vi "SV TDMS Write Y Properties.vi"(0 "tdms file":refnum<k34>, 1 "y-axis label":string, 2 "y-unit string":string, 5 "group name":string, 7 "channel name":string, 11 "error in (no error)":errorcluster, 12 "xchannel name":string) -> (4 "tdms file out":refnum<k34>, 6 "group name":string, 8 "channel name":string, 15 "error out":errorcluster)   [LabVIEW 2017]
uses:
  <vilib>/addons/_NISVFA/_Shared subVIs/Controls/NI Channel Properties.ctl
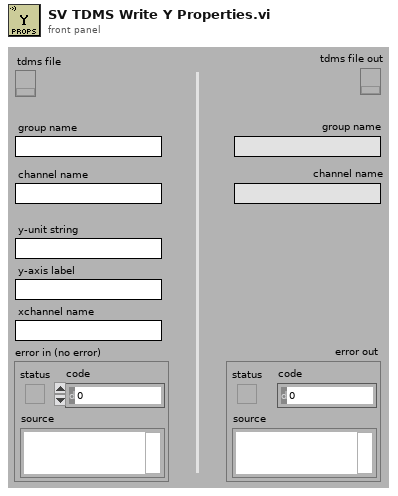
[diagram p1: front panel]
types:
  T1 = typedef "NI Channel Properties.ctl" = u16
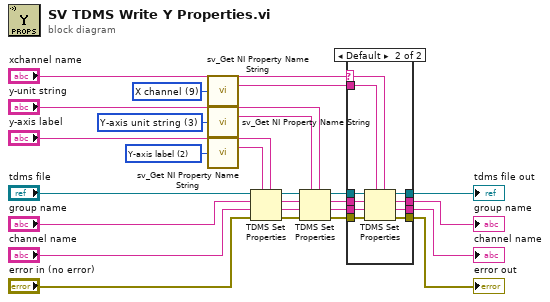
[diagram p0: block diagram]
diagram:
  w11 = T1 9 items=["Channel name", "Channel description", "Y-axis label", "Y-axis unit string", "X-axis label", "X-axis unit string", "x0", "dx", "Number of samples", "X channel", "Filter settled", "dB reference", "Window", "Window parameter", "Window size", "FFT size", "Peak units", "Spectrum type", "Magnitude scale", "Spectral density", "Sensor sensitivity (mV/EU)", "X-axis dimension", "LabVIEW datatype", "Function type", "Function subtype", "X-values"] ("property")
  w14 = T1 3 items=["Channel name", "Channel description", "Y-axis label", "Y-axis unit string", "X-axis label", "X-axis unit string", "x0", "dx", "Number of samples", "X channel", "Filter settled", "dB reference", "Window", "Window parameter", "Window size", "FFT size", "Peak units", "Spectrum type", "Magnitude scale", "Spectral density", "Sensor sensitivity (mV/EU)", "X-axis domain", "LabVIEW datatype"] ("property")
  w15 = T1 2 items=["Channel name", "Channel description", "Y-axis label", "Y-axis unit string", "X-axis label", "X-axis unit string", "x0", "dx", "Number of samples", "X channel", "Filter settled", "dB reference", "Window", "Window parameter", "Window size", "FFT size", "Peak units", "Spectrum type", "Magnitude scale", "Spectral density", "Sensor sensitivity (mV/EU)", "X-axis domain", "LabVIEW datatype"] ("property")
  n1 = call <vilib>:"sv_Get NI Property Name String.vi"("property"=w11) -> ("TDMS property name"=w10:string)  [unwired: 13 in, 1 out]
  n2 = call <vilib>:"sv_Get NI Property Name String.vi"("property"=w14) -> ("TDMS property name"=w13:string)  [unwired: 13 in, 1 out]
  n3 = call <vilib>:"sv_Get NI Property Name String.vi"("property"=w15) -> ("TDMS property name"=w12:string)  [unwired: 13 in, 1 out]
  n4 = TDMS Set Properties(5:"y-axis label", 7:w12, 8:"error in (no error)", 9:"channel name", 10:"group name", 11:"tdms file") -> (0:w16:errorcluster, 1:w23:string, 2:w22:string)  [unwired: 1 out]
  n5 = TDMS Set Properties(5:"y-unit string", 7:w13, 8:w16, 9:w23, 10:w22, 11:"tdms file") -> (0:w3:errorcluster, 1:w4:string, 2:w5:string, 3:w6:refnum<k34>)
  n6 = case shown="Default" "xchannel name" {
    selector: "xchannel name" -> [_ w29]
    tunnel: w10 -> [_ w38]
    tunnel: [w28 w37] -> w9
    tunnel: [w27 w36] -> w8
    tunnel: [w25 w35] -> w7
    tunnel: w6 -> [w28 w34]
    tunnel: w5 -> [w27 w33]
    tunnel: w4 -> [w26 w32]
    tunnel: w3 -> [w25 w31]
    tunnel: [w26 w30] -> w2
    frame "" {
    }
    frame Default {
      n7 = TDMS Set Properties(5:w29, 7:w38, 8:w31, 9:w32, 10:w33, 11:w34) -> (0:w35:errorcluster, 1:w30:string, 2:w36:string, 3:w37:refnum<k34>)
    }
  }
  "group name" <- w8
  "error out" <- w7
  "tdms file out" <- w9
  "channel name" <- w2
